vi "Path Manager.vi"(0 "Main File Path":path, 11 "Error IN":errorcluster) -> (4 "Path Location Cluster":T1, 15 "Error OUT":errorcluster)   [LabVIEW 2011]
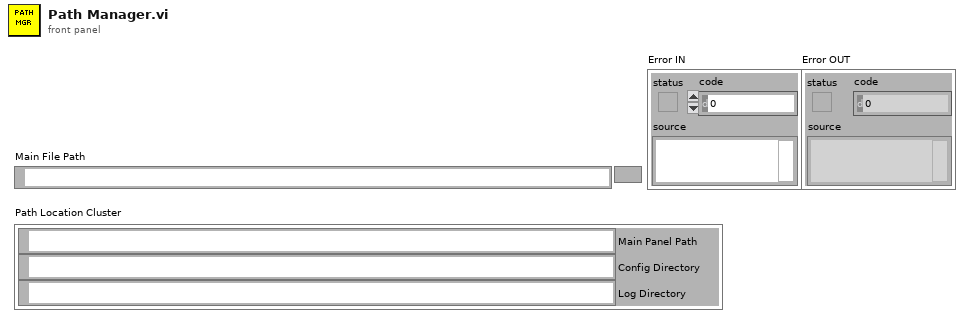
[diagram p1: front panel]
types:
  T1 = cluster{"Main Panel Path":path, "Config Directory":path, "Log Directory":path}
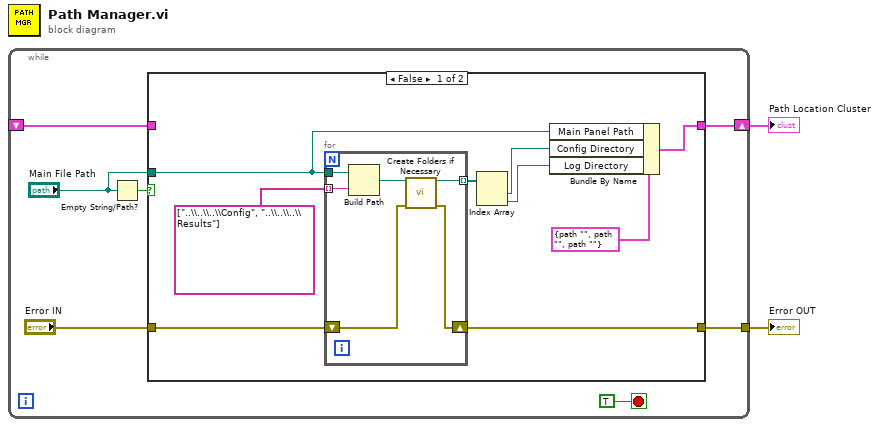
[diagram p0: block diagram]
diagram:
  n1 = while {
    shift-right: [w8] -> w2
    shift-left: _ -> [w7]
    tunnel: [w6] -> w1
    stop <- TRUE stop-if-true
    n2 = Empty String/Path?(string/path="Main File Path") -> (empty?=w4:bool)
    n3 = case shown="False" w4 {
      tunnel: [w17 w26] -> w8
      tunnel: w7 -> [_ w26]
      tunnel: [w11 w25] -> w6
      tunnel: "Error IN" -> [w16 w25]
      tunnel: "Main File Path" -> [w10 _]
      frame False {
        n4 = for {
          tunnel: w10 -> [w24]
          shift-right: [w21] -> w11
          shift-left: w16 -> [w22]
          tunnel: [w20] -> w14 mode=indexing
          tunnel: string[] ["..\\..\\..\\Config", "..\\..\\..\\Results"] -> [w19] mode=indexing
          n5 = Build Path(base path=w24, name or relative path=w19) -> (appended path=w23:path)
          n6 = call "Create Folders if Necessary.vi"("Report Directory IN"=w23, "Error IN"=w22) -> ("Report Directory OUT"=w20:path, "Error OUT"=w21:errorcluster)  [unwired: 12 in]
        }
        n7 = Index Array(array=w14) -> (element #1=w13:path, element #2=w12:path)  [unwired: 2 in]
        n8 = Bundle By Name(cluster=T1 {"Main Panel Path"=path "", "Config Directory"=path "", "Log Directory"=path ""} ("Path Location Cluster"), "Main Panel Path"=w10, "Config Directory"=w13, "Log Directory"=w12) -> (w17:T1)
      }
      frame True {
      }
    }
  }
  "Path Location Cluster" <- w2
  "Error OUT" <- w1
